vi "OLD_XLIN1.7-2048SQ TE0_Target.vi"() -> ()   [LabVIEW 2018]
uses:
  <vilib>/Platform/TimedLoop/XDataNode/timing_clust.ctl
  <vilib>/Platform/TimedLoop/XDataNode/nitl_modes.ctl
  <vilib>/Platform/TimedLoop/XDataNode/wakeup.ctl
  <vilib>/rvi/eio/common/nirviEmuTemplateMethod_errors.vi
  <vilib>/rvi/Emulation/niFpgaGetClockAttributes.vi
  <vilib>/rvi/Emulation/niFpgaSctlEmulationGetInTimedLoop.vi
  <vilib>/rvi/Emulation/niFpgaEmulationReportErrorSimple.vi
  <vilib>/rvi/Emulation/niFpgaProcessEmulError.vi
  <vilib>/rvi/Emulation/niFpgaCriticalErrorInLSC.vi
  <vilib>/rvi/interface/RandomDataEmulation/niFpgaRandomDataHandleErrors.vi
  <vilib>/eio/EIONode/EIONode.xnode
  <vilib>/Platform/TimedLoop/XDataNode/XDataNode.xnode
  <vilib>/rvi/DataTransferAndStorage/Container/XNode/niFpgaContainer.xnode
  <vilib>/rvi/interface/RandomDataEmulation/nirviRandomDataFpgaReadWriteTemplate.vi
  <vilib>/Platform/TimedLoop/XDataNode/XDNodeRunTimeDep.lvlib
panel:
  in  "Supply Select":u8(ring) items=["Local", "External"]
  in  "Falling CLK_3 = 1":u8=1
  in  "Rising CLK_4 = 2":u8=2
  in  "Counter R&F CLK_2 = 4":u8=4
  in  "F(F)/R(T)_FIFO":bool=TRUE
  in  "F(F)/R(T)_CmAD":bool
  in  "Falling CLK_7 = 1":u8=1
  in  "Rising CLK_7 = 1":u8=1
  in  "Falling CLK_6 = 2":u8=2
  in  "Rising CLK_6 = 2":u8=2
  in  "Counter R&F CLK_1 = 7":u8=7
  in  "Falling CLK_4 = 3":u8=3
  in  "Rising CLK_3 = 1":u8=1
  in  "Falling CLK_5 = 2":u8=2
  in  "Rising CLK_5 = 2":u8=2
  in  "Falling CLK_2 = 2":u8=2
  in  "Rising CLK_2 = 1":u8=1
  in  "Falling CLK_1 = 1":u8=1
  in  "Rising CLK_1 = 0":u8
  in  "Counter R CLK = 2":u8=2
  in  "ResetSetReg":bool
  in  "ResetSendData":bool
  out "SetRegIsDone":bool
  in  "Этап прошивки":T1(ring)
  in  "ResetFIFO":bool
  in  "Data Sample End":u8[](array[numeric])=[0, 5, 1, 0, 0]
  in  "Command End Readout":u8[](array[numeric])=[8, 4, 2, 0, 0]
  in  "Data Sample Start":u8[](array[numeric])=[0, 0, 1, 11, 1, 0, 0, 0, 0, 6, 0, 0, 15, 0, 1, 1, 5, 13, 13, 0]
  in  "Command Start Readout":u8[](array[numeric])=[8, 4, 2, 2, 2, 2, 9, 2, 2, 2, 2, 2, 2, 1, 1, 1, 1, 1, 1, 0]
  in  "Data Hold":u8[](array[numeric])=[0, 0, 0, 1, 1, 0, 0, 0, 5, 1, 0, 0, 0, 0, 0, 0, 0, 0, 0, 0, 3, 1, 0, 0, 1, 5, 1, 0, 0, 1, 3, 1, 0, 0, 1, 3, 1, 0, 0, 1, 11, 1, 11, 0, 1, 11, 1, 3, 0, 0, 0]
  in  "Command Start Integration":u8[](array[numeric])=[8, 4, 2, 2, 2, 2, 9, 2, 2, 2, 2, 2, 0, 0, 0, 0, 0, 8, 4, 2, 2, 2, 2, 9, 2, 2, 2, 2, 9, 2, 2, 2, 2, 9, 2, 2, 2, 2, 9, 2, 2, 2, 2, 9, 2, 2, 2, 2, 9, 0, 0]
  in  "SetReg":bool
  in  "Data Reset":u8[](array[numeric])=[0, 0, 0, 5, 0, 0, 0, 0, 0]
  in  "Command Reset":u8[](array[numeric])=[8, 4, 2, 2, 2, 2, 9, 0, 0]
  in  "IN1":bool
  in  "IN2":bool
  in  "RS":bool
  in  "1032 pixels":u16=1032
  out "FIFOIsDone":bool
  in  "R ADCCLK = 5":u16=5
  in  "R MCLK = 2":u16=2
  in  "FrameToFIFO":bool
  in  "Command array":bool[](array[boolean])=[FALSE, FALSE, FALSE, FALSE, FALSE, FALSE, FALSE, FALSE, FALSE, FALSE, FALSE, FALSE, FALSE, FALSE, FALSE, FALSE, FALSE]
  in  "Read(T)/Write(F)":bool
  in  "Enum":T2(ring)=enum."GREEN PGA"
  in  "Write Data":bool[](array[boolean])=[FALSE, FALSE, FALSE, FALSE, FALSE, FALSE, FALSE, FALSE, FALSE]
  out "READ":bool[](array[boolean])
  in  "Конфигурация":bool
  out "SendDataIsDone":bool
  in  "NumberOfAddFIFO":u16=2064
  in  "7..0(F)/0..7(T)":bool
  out "FIFOCounter":u16
  in  "CSTop":bool
  in  "ArraySize":u8=51
  in  "Command":u8[](array[numeric])=[8, 4, 2, 2, 2, 2, 2, 2, 2, 2, 2, 2, 2, 2, 2, 2, 2, 2, 2, 2, 2, 2, 2, 2, 2, 2, 2, 2, 2, 2, 2, 2, 2, 8, 4, 1, 1, 1, 1, 1, 1, 1, 1, 1, 0, 0, 0, 0, 0, 0, 0]
  in  "Data":u8[](array[numeric])=[0, 9, 12, 11, 0, 6, 0, 2, 11, 0, 8, 0, 0, 0, 0, 9, 1, 3, 3, 7, 15, 15, 5, 15, 0, 1, 15, 15, 5, 8, 5, 2, 3, 0, 8, 2, 3, 3, 3, 3, 3, 3, 3, 2, 0, 0, 0, 0, 0, 0, 0]
  in  "Data CSBot":u8[](array[numeric])=[0, 9, 8, 11, 0, 6, 0, 2, 11, 0, 8, 0, 0, 0, 0, 9, 1, 3, 11, 7, 15, 15, 5, 15, 0, 1, 15, 15, 5, 8, 5, 2, 3, 0, 8, 2, 3, 3, 3, 3, 3, 3, 3, 2, 0]
  in  "CSBot":bool
  in  "Автомат":bool
  in  "Data CSTop":u8[](array[numeric])=[0, 9, 12, 11, 0, 6, 0, 2, 11, 0, 8, 0, 0, 0, 0, 9, 1, 3, 3, 7, 15, 15, 5, 15, 0, 1, 15, 15, 5, 8, 5, 2, 3, 0, 8, 2, 3, 3, 3, 3, 3, 3, 3, 2, 0]
  in  "Command CS":u8[](array[numeric])=[8, 4, 2, 2, 2, 2, 2, 2, 2, 2, 2, 2, 2, 2, 2, 2, 2, 2, 2, 2, 2, 2, 2, 2, 2, 2, 2, 2, 2, 2, 2, 2, 2, 8, 4, 1, 1, 1, 1, 1, 1, 1, 1, 1, 0]
  in  "Stop_FPGA":bool
  in  "SendData":bool
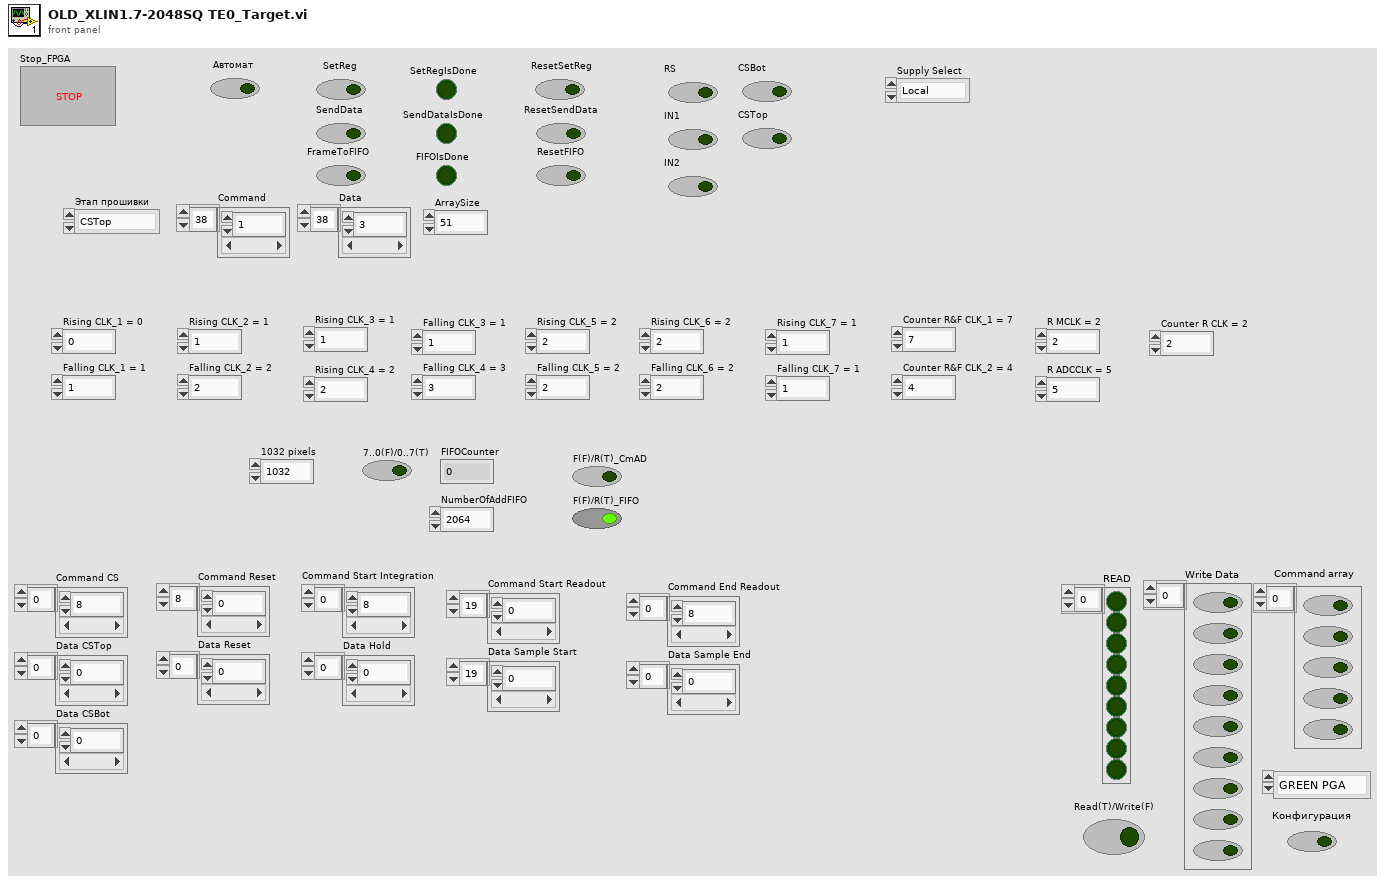
[diagram p1: front panel]
types:
  T1 = enum16{"CSTop", "CSBot", "Reset", "Hold", "Sample Start", "Sample End"}
  T2 = enum16{"Configuration", "MUX", "RED PGA", "GREEN PGA", "BLUE PGA", "RED OFF", "GREEN OFF", "BLUE OFF"}
  T3 = typedef "XDNodeRunTimeDep.lvlib/timing_clust.ctl" = cluster{"Expected End [f-1]":u64, "Actual End [f-1]":u64, "Finished Late? [f-1]":bool, "Expected End [i-1]":u64, "Actual End [i-1]":u64, "Finished Late? [i-1]":bool, "Expected Start [i]":u64, "Actual Start [i]":u64, "Expected Start [f]":u64, "Actual Start [f]":u64, "Source Name":string, "Structure Name":string, "Period":i64, "Deadline":i64, "Offset":i64, "Start":i64, "Priority":i32, "Timeout":i32, "Mode":T4, "Wakeup Reason":T5, "Error":errorcluster, "Source Type":string, "Secondary Source Type":string, "Global End Time":u64, "Global Start Time":u64, "Frame Duration":u64, "Iteration Duration":u64, "Assigned CPU":i32, "I/O Scan Engine Mode":u32}
  T4 = typedef "XDNodeRunTimeDep.lvlib/nitl_modes.ctl" = enum32{"No Change", "Process missed periods, maintain original phase", "Discard missed periods, maintain original phase", "Process missed periods, ignore original phase", "Discard missed periods, ignore original phase"}
  T5 = typedef "XDNodeRunTimeDep.lvlib/wakeup.ctl" = enum32{"Normal", "Aborted", "Asynchronous wakeup", "Timing source error", "Timed loop error", "Timeout"}
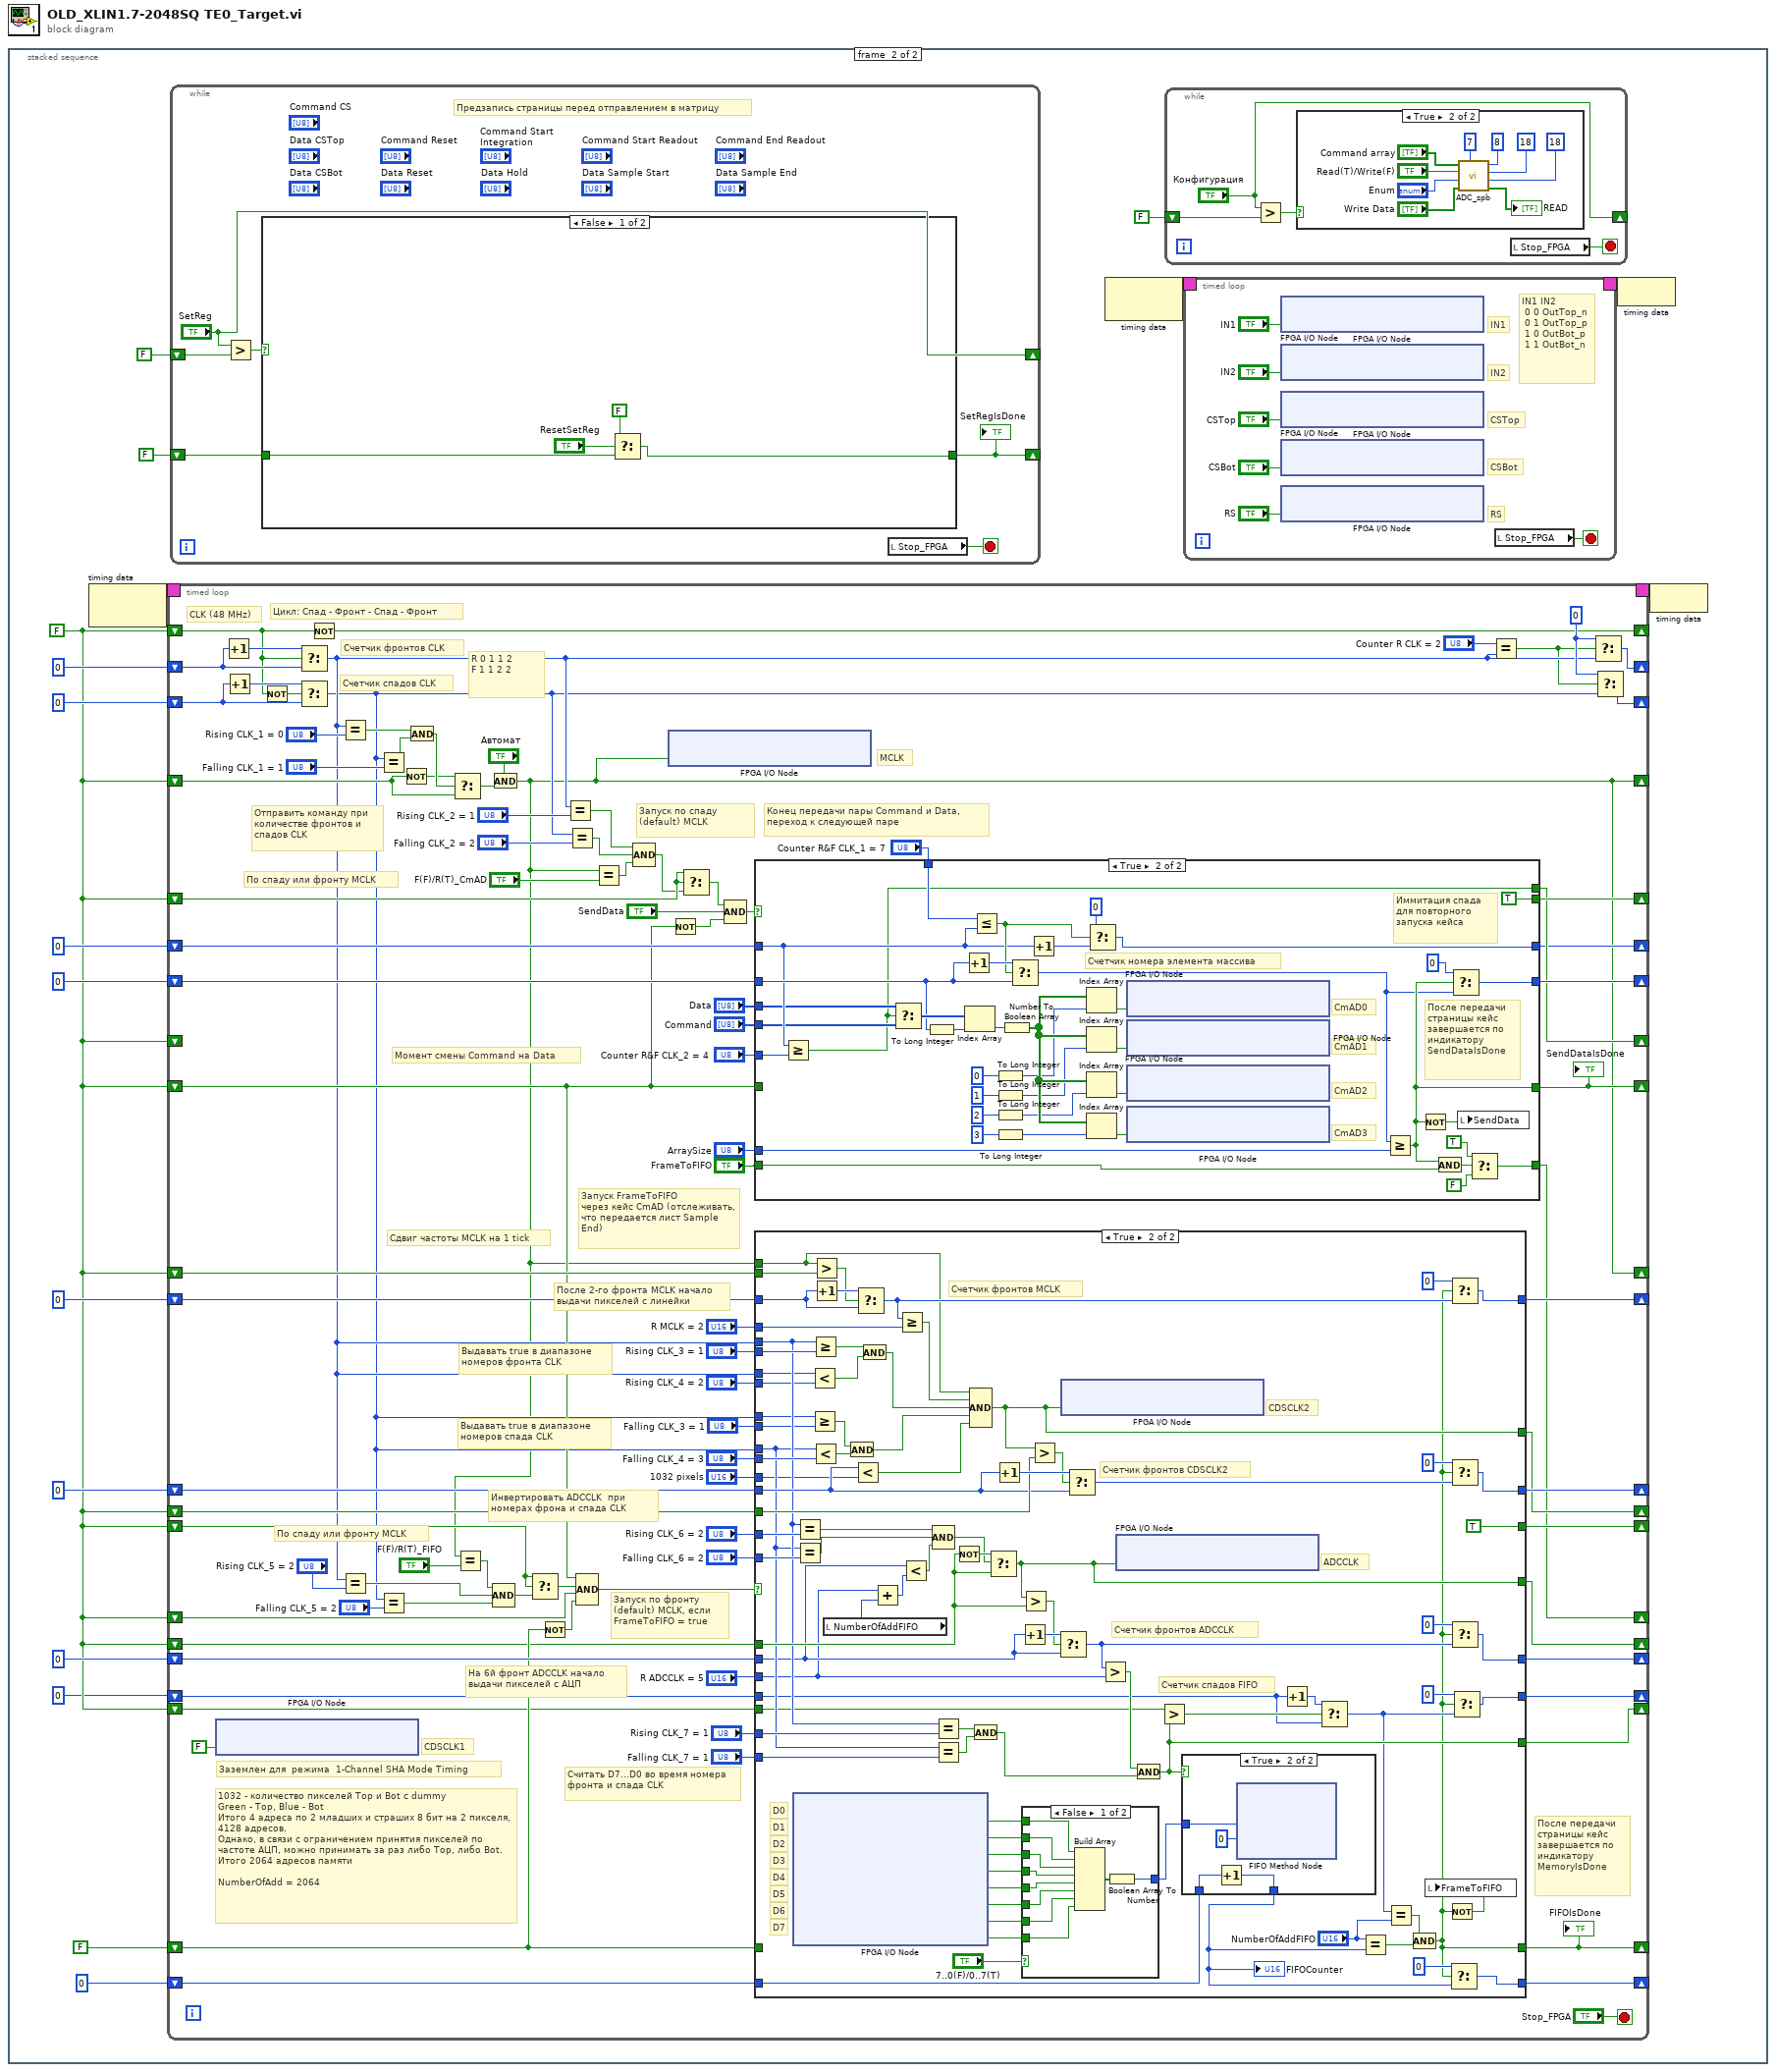
[diagram p0: block diagram]
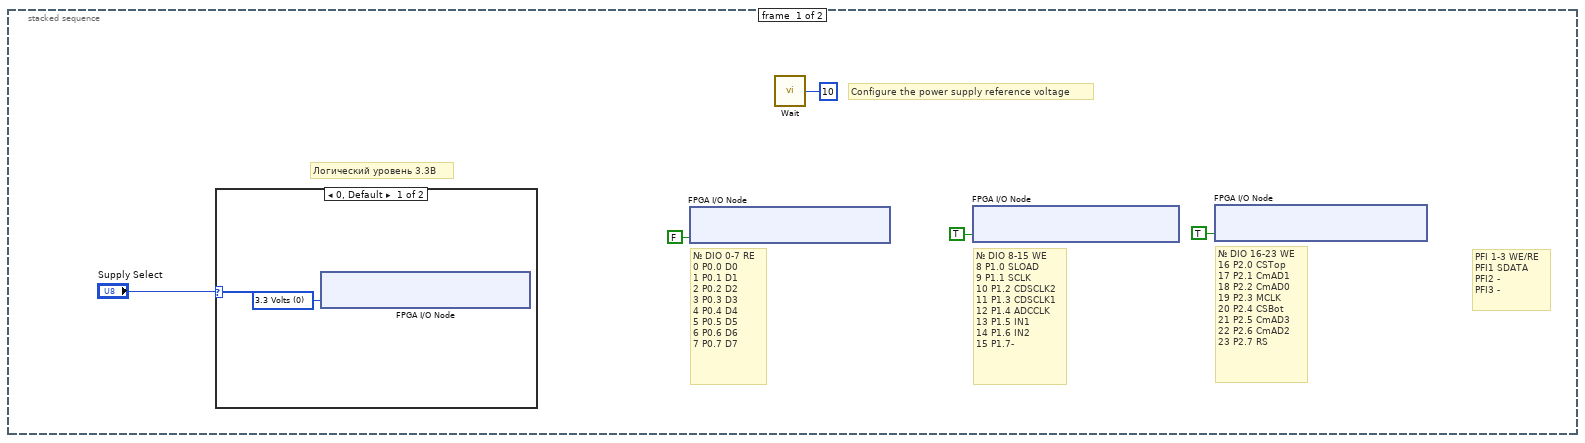
[diagram p2: hidden frame]
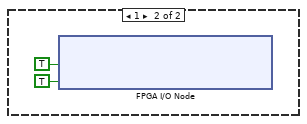
[diagram p3: hidden frame]
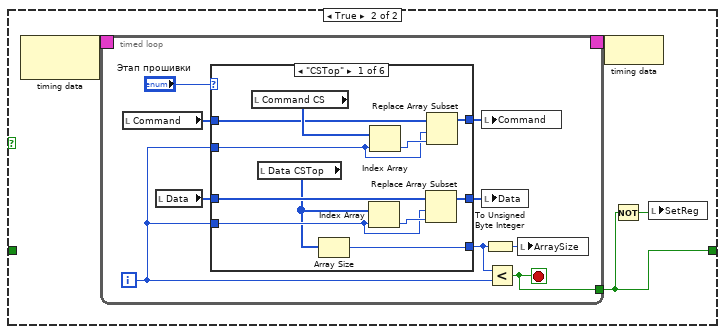
[diagram p4: hidden frame]
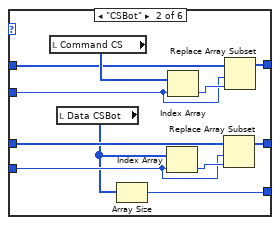
[diagram p5: hidden frame]
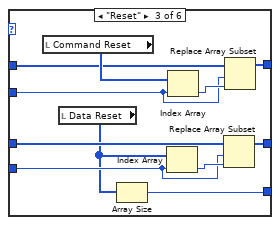
[diagram p6: hidden frame]
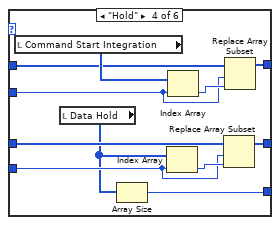
[diagram p7: hidden frame]
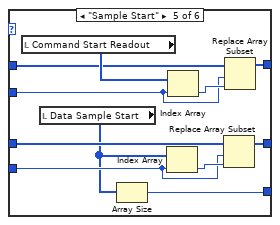
[diagram p8: hidden frame]
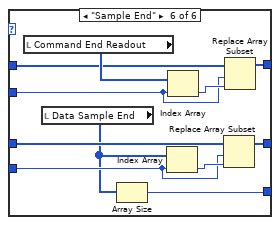
[diagram p9: hidden frame]
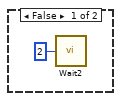
[diagram p10: hidden frame]
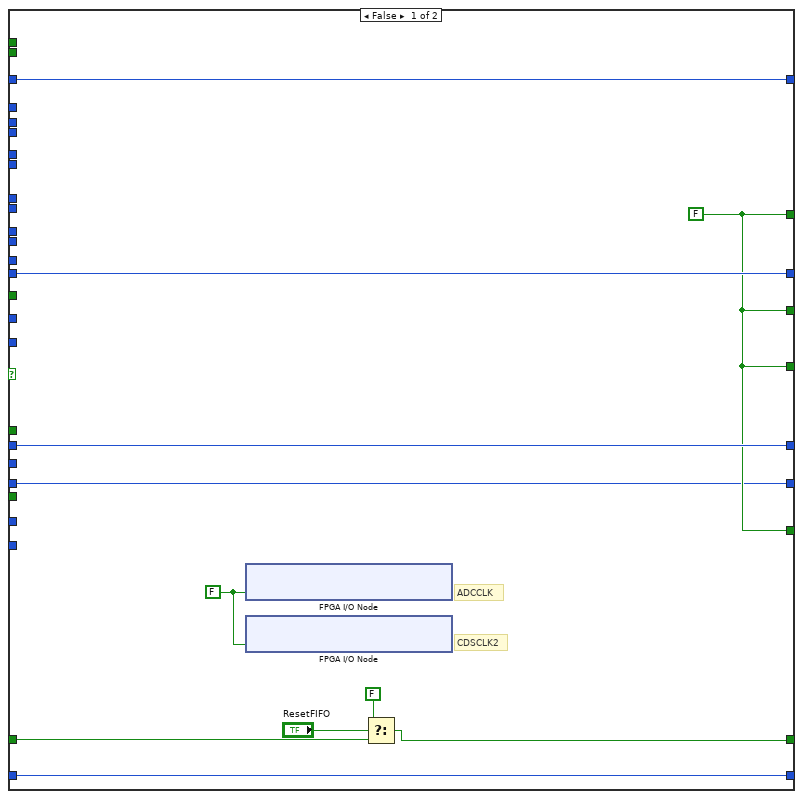
[diagram p11: hidden frame]
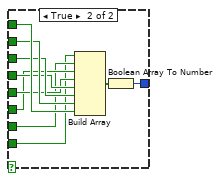
[diagram p12: hidden frame]
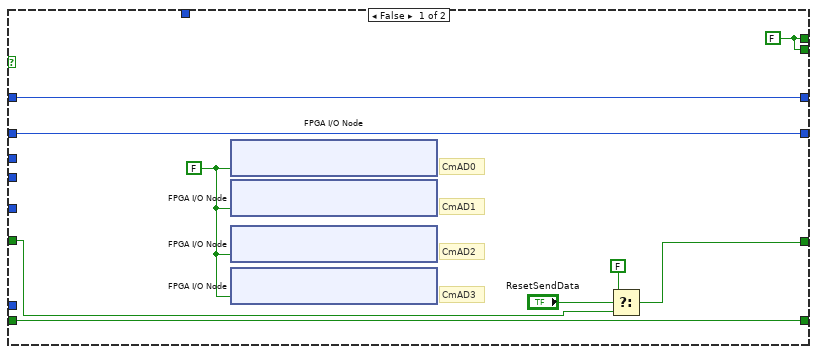
[diagram p14: hidden frame]
diagram:
  n1 = stacked-sequence {
    frame #0 {
      # "Логический уровень 3.3В"
      # "№\tDIO 16-23\tWE\n16\tP2.0\tCSTop\n17\tP2.1\tCmAD1\n18\tP2.2\tCmAD0\n19\tP2.3\tMCLK\n20\tP2.4\tCSBot\n21\tP2.5\tCmAD3\n22\tP2.6\tCmAD2\n23\tP2.7\tRS"
      # "№\tDIO 8-15\tWE\n8\tP1.0\tSLOAD\n9\tP1.1\tSCLK\n10\tP1.2\tCDSCLK2\n11\tP1.3\tCDSCLK1\n12\tP1.4\tADCCLK\n13\tP1.5\tIN1\n14\tP1.6\tIN2\n15\tP1.7-"
      # "PFI 1-3\tWE/RE\nPFI1\tSDATA\nPFI2\t-\nPFI3\t-"
      # "№\tDIO 0-7\tRE\n0\tP0.0\tD0\n1\tP0.1\tD1\n2\tP0.2\tD2\n3\tP0.3\tD3\n4\tP0.4\tD4\n5\tP0.5\tD5\n6\tP0.6\tD6\n7\tP0.7\tD7"
      # "Configure the power supply reference voltage"
      n2 = case shown="0, Default" "Supply Select" {
        frame 0, Default {
          w6 = u8 0 items=["3.3 Volts", "2.5 Volts", "1.8 Volts"] ("Internal Power Supply Voltage")
          n3 = xnode "FPGA I/O Node"("IO Module\\Local_Supply_Select"=w6) -> ()  [unwired: 1 in, 1 out]
        }
        frame 1 {
          n4 = xnode "FPGA I/O Node"("IO Module\\DDCA_Supply_Select"=TRUE ("IO Module\\DDCA_Supply_Select"), "IO Module\\DDCB_Supply_Select"=TRUE ("IO Module\\DDCB_Supply_Select")) -> ()  [unwired: 2 in, 2 out]
        }
      }
      n5 = xnode "FPGA I/O Node"("IO Module\\DDCA_DIO0-7_WE"=FALSE ("IO Module\\DDCA_DIO0-7_WE")) -> ()  [unwired: 1 in, 1 out]
      n6 = call "Wait"("Count(mSec)"=u8 10) -> ()  [unwired: 1 out]
      n7 = xnode "FPGA I/O Node"("IO Module\\DDCA_DIO8-15_WE"=TRUE ("IO Module\\DDCA_DIO8-15_WE")) -> ()  [unwired: 1 in, 1 out]
      n8 = xnode "FPGA I/O Node"("IO Module\\DDCA_DIO16-23_WE"=TRUE ("IO Module\\DDCA_DIO16-23_WE")) -> ()  [unwired: 1 in, 1 out]
    }
    frame #1 {
      w10 = FALSE
      n9 = node-c288() -> (w26:T3)  [unwired: 1 in]
      n10 = timed-loop {
        timing: w26 -> [_]
        timing-out: [_] -> w25
        shift-right: [w146] -> _
        shift-left: w10 -> [w209]
        shift-right: [w235] -> _
        shift-left: u8 0 -> [w239]
        shift-right: [w234] -> _
        shift-left: w10 -> [w220]
        shift-right: [w233] -> _
        shift-left: u16 0 -> [w232]
        shift-right: [w230] -> _
        shift-left: u16 0 -> [w231]
        shift-right: [w228] -> _
        shift-left: u16 0 -> [w229]
        shift-right: [w226] -> _
        shift-left: u16 0 -> [w227]
        shift-right: [w225] -> _
        shift-left: w10 -> [w176]
        shift-right: [w224] -> _
        shift-left: FALSE ("IO Module\\DDCA_DIO11_Write") -> [w212]
        shift-right: [w153] -> _
        shift-left: w10 -> [w152]
        shift-right: [w223] -> _
        shift-left: w10 -> [w163]
        shift-right: [w217] -> _
        shift-left: w10 -> [w218]
        shift-right: [w213] -> _
        shift-left: w10 -> [w172]
        shift-right: [w205] -> _
        shift-left: u8 0 -> [w198]
        shift-right: [w206] -> _
        shift-left: u8 0 -> [w199]
        shift-right: [w184] -> _
        shift-left: w10 -> [_]
        shift-right: [w182] -> _
        shift-left: u8 0 -> [w183]
        shift-right: [w146] -> _
        shift-left: w10 -> [w180]
        shift-right: [w171] -> _
        shift-left: w10 -> [w173]
        shift-right: [w159] -> _
        shift-left: w10 -> [w160]
        shift-right: [w157] -> _
        shift-left: u16 0 -> [w158]
        stop <- "Stop_FPGA" stop-if-true
        w204 = u8 0 ("f")
        # "Цикл: Спад - Фронт - Спад - Фронт"
        # "Конец передачи пары Command и Data, переход к следующей паре"
        # "Запуск по спаду (default) MCLK"
        # "Момент смены Command на Data"
        # "По спаду или фронту MCLK"
        # "Считать D7...D0 во время номера фронта и спада CLK"
        # "Инвертировать ADCCLK  при номерах фрона и спада CLK"
        # "Выдавать true в диапазоне номеров спада CLK"
        # "Выдавать true в диапазоне номеров фронта CLK"
        # "По спаду или фронту MCLK"
        # "Заземлен для  режима  1-Channel SHA Mode Timing"
        # "CDSCLK1"
        # "R 0 1 1 2\nF 1 1 2 2"
        # "Счетчик спадов CLK"
        # "Счетчик фронтов CLK"
        # "После 2-го фронта MCLK начало выдачи пикселей с линейки"
        # "На 6й фронт ADCCLK начало выдачи пикселей с АЦП"
        # "Отправить команду при количестве фронтов и спадов CLK"
        # "После передачи страницы кейс завершается по индикатору MemoryIsDone"
        # "Запуск FrameToFIFO\nчерез кейс CmAD (отслеживать, что передается лист Sample End)"
        # "CLK (48 MHz)"
        # "1032 - количество пикселей Top и Bot с dummy\nGreen - Top, Blue - Bot\nИтого 4 адреса по 2 младших и страших 8 бит на 2 пикселя, 4128 адресов.\nОднако, в связи с ограничением принятия пикселей по частоте АЦП, можно принимать за раз либо Top, либо Bot. Итого 2064 адресов памяти\n\nNumberOfAdd = 2064"
        # "Сдвиг частоты MCLK на 1 tick"
        # "Запуск по фронту (default) MCLK, если FrameToFIFO = true"
        # "MCLK"
        n11 = xnode "FPGA I/O Node"("IO Module\\DDCA_DIO11_Write"=FALSE ("IO Module\\DDCA_DIO11_Write")) -> ()  [unwired: 1 in, 1 out]
        n12 = Increment(x=w199) -> (x+1=w208:u8)
        n13 = Increment(x=w198) -> (x+1=w207:u8)
        n14 = Not(x=w152) -> (.not. x?=w210:bool)
        n15 = Select(t=w208, s=w152, f=w199) -> (s? t:f=w150:u8)
        n16 = Select(t=w207, s=w210, f=w198) -> (s? t:f=w149:u8)
        n17 = Not(x=w152) -> (.not. x?=w153:bool)
        n18 = Equal?(x=w150, y="Rising CLK_1 = 0") -> (x = y?=w203:bool)
        n19 = Equal?(x=w150, y="Rising CLK_5 = 2") -> (x = y?=w179:bool)
        n20 = Equal?(x=w149, y="Falling CLK_1 = 1") -> (x = y?=w200:bool)
        n21 = Equal?(x=w149, y="Falling CLK_5 = 2") -> (x = y?=w178:bool)
        n22 = Not(x=w209) -> (.not. x?=w147:bool)
        n23 = And(x=w203, y=w200) -> (x .and. y?=w197:bool)
        n24 = Select(t=w147, s=w197, f=w209) -> (s? t:f=w222:bool)
        n25 = And(x="Автомат", y=w222) -> (x .and. y?=w146:bool)
        n26 = Equal?(x=w146, y="F(F)/R(T)_FIFO") -> (x = y?=w165:bool)
        n27 = Compound Arithmetic op=AND(w165, w179, w178) -> (w177:bool)
        n28 = Select(t=w218, s=w218, f=w177) -> (s? t:f=w162:bool)
        n29 = Not(x=w212) -> (.not. x?=w170:bool)
        n30 = Equal?(x=w150, y="Rising CLK_2 = 1") -> (x = y?=w189:bool)
        n31 = Equal?(x=w149, y="Falling CLK_2 = 2") -> (x = y?=w188:bool)
        n32 = Compound Arithmetic op=AND(w163, w162, w172, w170) -> (w219:bool)
        n33 = Equal?(x=w146, y="F(F)/R(T)_CmAD") -> (x = y?=w187:bool)
        n34 = Compound Arithmetic op=AND(w189, w188, w187) -> (w144:bool)
        n35 = xnode "FPGA I/O Node"("IO Module\\DDCA_DIO19_Write"=w146) -> ()  [unwired: 1 in, 1 out]
        n36 = Not(x=w163) -> (.not. x?=w216:bool)
        n37 = Select(t=w220, s=w220, f=w144) -> (s? t:f=w221:bool)
        n38 = Compound Arithmetic op=AND(w221, "SendData", w216) -> (w145:bool)
        n39 = case shown="True" w145 {
          tunnel: w239 -> [w365 w388]
          tunnel: "ArraySize" -> [_ w387]
          tunnel: [w365 w384] -> w235
          tunnel: "FrameToFIFO" -> [w366 w400]
          tunnel: [w363 TRUE] -> w234
          tunnel: [w367 w383] -> w223
          tunnel: w163 -> [w368 _]
          tunnel: [w366 w385] -> w213
          tunnel: "Command" -> [_ w373]
          tunnel: "Data" -> [_ w372]
          tunnel: [w363 w371] -> w184
          tunnel: w183 -> [w364 w374]
          tunnel: [w364 w377] -> w182
          tunnel: "Counter R&F CLK_1 = 7" -> [_ w378]
          tunnel: "Counter R&F CLK_2 = 4" -> [_ w375]
          frame False {
            w362 = FALSE ("t")
            w363 = FALSE
            # "CmAD3"
            # "CmAD2"
            # "CmAD1"
            # "CmAD0"
            n40 = xnode "FPGA I/O Node"("IO Module\\DDCA_DIO18_Write"=w362) -> ()  [unwired: 1 in, 1 out]
            n41 = xnode "FPGA I/O Node"("IO Module\\DDCA_DIO17_Write"=w362) -> ()  [unwired: 1 in, 1 out]
            n42 = xnode "FPGA I/O Node"("IO Module\\DDCA_DIO22_Write"=w362) -> ()  [unwired: 1 in, 1 out]
            n43 = xnode "FPGA I/O Node"("IO Module\\DDCA_DIO21_Write"=w362) -> ()  [unwired: 1 in, 1 out]
            n44 = Select(t=FALSE, s="ResetSendData", f=w368) -> (s? t:f=w367:bool)
          }
          frame True {
            # "Иммитация спада для повторного запуска кейса"
            # "После передачи страницы кейс завершается по индикатору SendDataIsDone"
            # "Счетчик номера элемента массива"
            # "CmAD3"
            # "CmAD2"
            # "CmAD1"
            # "CmAD0"
            n45 = Greater Or Equal?(x=w374, y=w375) -> (x >= y?=w371:bool)
            n46 = Select(t=w372, s=w371, f=w373) -> (s? t:f=w408:u8[])
            n47 = To Long Integer(number=w388) -> (32bit integer=w407:i32)
            n48 = Increment(x=w388) -> (x+1=w410:u8)
            n49 = Index Array(array=w408, index=w407) -> (element=w409:u8)
            n50 = Less Or Equal?(x=w378, y=w374) -> (x <= y?=w380:bool)
            n51 = To Long Integer(number=u8 0 ("CmAD0_bit_0")) -> (32bit integer=w393:i32)
            n52 = To Long Integer(number=u8 1 ("CmAD1_bit_1")) -> (32bit integer=w392:i32)
            n53 = To Long Integer(number=u8 2 ("CmAD2_bit_2")) -> (32bit integer=w391:i32)
            n54 = To Long Integer(number=u8 3 ("CmAD3_bit_3")) -> (32bit integer=w389:i32)
            n55 = Number To Boolean Array(number=w409) -> (Boolean array=w405:bool[])
            n56 = Select(t=w410, s=w380, f=w388) -> (s? t:f=w382:u8)
            n57 = Increment(x=w374) -> (x+1=w376:u8)
            n58 = Index Array(array=w405, index=w393) -> (element=w406:bool)
            n59 = Index Array(array=w405, index=w392) -> (element=w402:bool)
            n60 = Index Array(array=w405, index=w391) -> (element=w404:bool)
            n61 = Index Array(array=w405, index=w389) -> (element=w403:bool)
            n62 = Select(t=u8 0, s=w380, f=w376) -> (s? t:f=w377:u8)
            n63 = xnode "FPGA I/O Node"("IO Module\\DDCA_DIO18_Write"=w406) -> ()  [unwired: 1 in, 1 out]
            n64 = xnode "FPGA I/O Node"("IO Module\\DDCA_DIO17_Write"=w402) -> ()  [unwired: 1 in, 1 out]
            n65 = xnode "FPGA I/O Node"("IO Module\\DDCA_DIO22_Write"=w404) -> ()  [unwired: 1 in, 1 out]
            n66 = xnode "FPGA I/O Node"("IO Module\\DDCA_DIO21_Write"=w403) -> ()  [unwired: 1 in, 1 out]
            n67 = Greater Or Equal?(x=w382, y=w387) -> (x >= y?=w383:bool)
            n68 = Not(x=w383) -> (.not. x?=w386:bool)
            n69 = And(x=w383, y=w400) -> (x .and. y?=w401:bool)
            n70 = Select(t=u8 0, s=w383, f=w382) -> (s? t:f=w384:u8)
            n71 = local write "SendData"(w386) -> ()
            n72 = Select(t=TRUE ("f"), s=w401, f=FALSE) -> (s? t:f=w385:bool)
          }
        }
        "SendDataIsDone" <- w223
        n73 = case shown="True" w219 {
          tunnel: [w246 w254] -> w233
          tunnel: w232 -> [w246 w326]
          tunnel: w231 -> [w244 w336]
          tunnel: [w244 w315] -> w230
          tunnel: w229 -> [w243 w281]
          tunnel: [w243 w308] -> w228
          tunnel: w227 -> [w245 w317]
          tunnel: [w245 w313] -> w226
          tunnel: w180 -> [_ w303]
          tunnel: w176 -> [_ w318]
          tunnel: [w241 w285] -> w225
          tunnel: [w248 w251] -> w224
          tunnel: w212 -> [w247 _]
          tunnel: [w241 TRUE ("f")] -> w217
          tunnel: "R MCLK = 2" -> [_ w283]
          tunnel: "1032 pixels" -> [_ w282]
          tunnel: "R ADCCLK = 5" -> [_ w278]
          tunnel: w150 -> [_ w292]
          tunnel: "Rising CLK_3 = 1" -> [_ w306]
          tunnel: w149 -> [_ w291]
          tunnel: "Falling CLK_4 = 3" -> [_ w305]
          tunnel: w146 -> [_ w261]
          tunnel: "Rising CLK_6 = 2" -> [_ w302]
          tunnel: "Falling CLK_6 = 2" -> [_ w301]
          tunnel: w173 -> [_ w298]
          tunnel: [w241 w284] -> w171
          tunnel: "Rising CLK_7 = 1" -> [_ w293]
          tunnel: "Falling CLK_7 = 1" -> [_ w294]
          tunnel: w160 -> [_ w276]
          tunnel: [w241 w275] -> w159
          tunnel: w158 -> [w240 w272]
          tunnel: [w240 w270] -> w157
          tunnel: "Rising CLK_4 = 2" -> [_ w264]
          tunnel: w150 -> [_ w263]
          tunnel: w149 -> [_ w256]
          tunnel: "Falling CLK_3 = 1" -> [_ w255]
          frame False {
            w242 = FALSE ("IO Module\\DDCA_DIO12_Write")
            w241 = FALSE
            # "CDSCLK2"
            # "ADCCLK"
            n74 = xnode "FPGA I/O Node"("IO Module\\DDCA_DIO12_Write"=w242) -> ()  [unwired: 1 in, 1 out]
            n75 = xnode "FPGA I/O Node"("IO Module\\DDCA_DIO10_Write"=w242) -> ()  [unwired: 1 in, 1 out]
            n76 = Select(t=FALSE, s="ResetFIFO", f=w247) -> (s? t:f=w248:bool)
          }
          frame True {
            # "Счетчик спадов FIFO"
            # "ADCCLK"
            # "Счетчик фронтов CDSCLK2"
            # "Счетчик фронтов ADCCLK"
            # "Счетчик фронтов MCLK"
            # "D7"
            # "D6"
            # "D5"
            # "D4"
            # "D3"
            # "D2"
            # "D1"
            # "D0"
            # "CDSCLK2"
            n77 = xnode "FPGA I/O Node"() -> ("IO Module\\DDCA_DIO0_Read"=w327:bool, "IO Module\\DDCA_DIO1_Read"=w328:bool, "IO Module\\DDCA_DIO2_Read"=w329:bool, "IO Module\\DDCA_DIO3_Read"=w330:bool, "IO Module\\DDCA_DIO4_Read"=w331:bool, "IO Module\\DDCA_DIO5_Read"=w332:bool, "IO Module\\DDCA_DIO6_Read"=w333:bool, "IO Module\\DDCA_DIO7_Read"=w334:bool)  [unwired: 8 in, 8 out]
            n78 = Equal?(x=w292, y=w302) -> (x = y?=w287:bool)
            n79 = Equal?(x=w291, y=w301) -> (x = y?=w289:bool)
            n80 = Less?(x=w263, y=w264) -> (x < y?=w262:bool)
            n81 = Greater Or Equal?(x=w256, y=w255) -> (x >= y?=w258:bool)
            n82 = Greater Or Equal?(x=w292, y=w306) -> (x >= y?=w265:bool)
            n83 = Less?(x=w291, y=w305) -> (x < y?=w304:bool)
            n84 = Greater?(x=w261, y=w303) -> (0:w321:bool)
            n85 = Increment(x=w336) -> (x+1=w324:u16)
            n86 = local read "NumberOfAddFIFO"() -> (w279:u16)
            n87 = And(x=w258, y=w304) -> (x .and. y?=w257:bool)
            n88 = Less?(x=w317, y=w282) -> (x < y?=w290:bool)
            n89 = Select(t=w324, s=w321, f=w336) -> (s? t:f=w286:u16)
            n90 = And(x=w265, y=w262) -> (x .and. y?=w259:bool)
            n91 = Add(x=w278, y=w279) -> (x+y=w277:u16)
            n92 = Greater Or Equal?(x=w286, y=w283) -> (x >= y?=w260:bool)
            n93 = Less?(x=w281, y=w277) -> (x < y?=w280:bool)
            n94 = Compound Arithmetic op=AND(w287, w289, w280) -> (w288:bool)
            n95 = Equal?(x=w292, y=w293) -> (x = y?=w297:bool)
            n96 = Equal?(x=w291, y=w294) -> (x = y?=w296:bool)
            n97 = Not(x=w298) -> (.not. x?=w300:bool)
            n98 = Compound Arithmetic op=AND(w261, w260, w259, w257, w290) -> (w285:bool)
            n99 = And(x=w297, y=w296) -> (x .and. y?=w295:bool)
            n100 = Select(t=w300, s=w288, f=w298) -> (s? t:f=w284:bool)
            n101 = Increment(x=w317) -> (x+1=w322:u16)
            n102 = Increment(x=w281) -> (x+1=w323:u16)
            n103 = Greater?(x=w284, y=w298) -> (0:w299:bool)
            n104 = case shown="False" "7..0(F)/0..7(T)" {
              tunnel: w327 -> [w346 w354]
              tunnel: w328 -> [w345 w353]
              tunnel: w329 -> [w344 w352]
              tunnel: w330 -> [w343 w351]
              tunnel: w331 -> [w342 w350]
              tunnel: w332 -> [w341 w349]
              tunnel: w333 -> [w340 w348]
              tunnel: w334 -> [w339 w347]
              tunnel: [w337 w355] -> w325
              frame False {
                n105 = Build Array(w346, w345, w344, w343, w342, w341, w340, w339) -> (w338:bool[])
                n106 = Boolean Array To Number(Boolean array=w338) -> (number=w337:u8)
              }
              frame True {
                n107 = Build Array(w347, w348, w349, w350, w351, w352, w353, w354) -> (w356:bool[])
                n108 = Boolean Array To Number(Boolean array=w356) -> (number=w355:u8)
              }
            }
            n109 = Greater?(x=w285, y=w318) -> (0:w319:bool)
            n110 = Select(t=w323, s=w299, f=w281) -> (s? t:f=w307:u16)
            n111 = xnode "FPGA I/O Node"("IO Module\\DDCA_DIO10_Write"=w285) -> ()  [unwired: 1 in, 1 out]
            n112 = Select(t=w322, s=w319, f=w317) -> (s? t:f=w312:u16)
            n113 = Greater?(x=w307, y=w278) -> (0:w320:bool)
            n114 = xnode "FPGA I/O Node"("IO Module\\DDCA_DIO12_Write"=w284) -> ()  [unwired: 1 in, 1 out]
            n115 = And(x=w320, y=w295) -> (x .and. y?=w275:bool)
            n116 = Greater?(x=w276, y=w275) -> (0:w274:bool)
            n117 = case shown="True" w275 {
              tunnel: [w357 w361] -> w253
              tunnel: w326 -> [w357 w360]
              tunnel: w325 -> [_ w358]
              frame False {
              }
              frame True {
                n118 = Increment(x=w360) -> (x+1=w361:u16)
                n119 = xnode ("FIFO Method Node")("Element"=w358, "Timeout"=0) -> ()  [unwired: 1 in, 2 out]
              }
            }
            "FIFOCounter" <- w253
            n120 = Increment(x=w272) -> (x+1=w273:u16)
            n121 = Select(t=w273, s=w274, f=w272) -> (s? t:f=w268:u16)
            n122 = Equal?(x="NumberOfAddFIFO", y=w253) -> (x = y?=w266:bool)
            n123 = Equal?(x=w268, y="NumberOfAddFIFO") -> (x = y?=w269:bool)
            n124 = Compound Arithmetic op=AND(w269, w266) -> (w251:bool)
            n125 = Not(x=w251) -> (.not. x?=w252:bool)
            n126 = local write "FrameToFIFO"(w252) -> ()
            n127 = Select(t=u16 0, s=w251, f=w253) -> (s? t:f=w254:u16)
            n128 = Select(t=u16 0, s=w251, f=w286) -> (s? t:f=w315:u16)
            n129 = Select(t=u16 0, s=w251, f=w312) -> (s? t:f=w313:u16)
            n130 = Select(t=u16 0, s=w251, f=w307) -> (s? t:f=w308:u16)
            n131 = Select(t=u16 0, s=w251, f=w268) -> (s? t:f=w270:u16)
          }
        }
        "FIFOIsDone" <- w224
        n132 = Equal?(x="Counter R CLK = 2", y=w150) -> (x = y?=w148:bool)
        n133 = Select(t=w204, s=w148, f=w150) -> (s? t:f=w206:u8)
        n134 = Select(t=w204, s=w148, f=w149) -> (s? t:f=w205:u8)
      }
      n135 = while {
        shift-right: ["SetReg"] -> _
        shift-left: FALSE -> [w41]
        shift-right: [w37] -> _
        shift-left: FALSE -> [w38]
        stop <- w42 stop-if-true
        # "Предзапись страницы перед отправлением в матрицу"
        n136 = Greater?(x="SetReg", y=w41) -> (0:w40:bool)
        n137 = case shown="False" w40 {
          tunnel: [w43 w47] -> w37
          tunnel: w38 -> [w45 _]
          frame False {
            n138 = Select(t=FALSE, s="ResetSetReg", f=w45) -> (s? t:f=w43:bool)
          }
          frame True {
            n139 = node-c288() -> (w50:T3)  [unwired: 1 in]
            n140 = timed-loop {
              timing: w50 -> [_]
              timing-out: [_] -> w49
              tunnel: [w53] -> w47
              i -> [w54]
              stop <- w53 stop-if-true
              n141 = local read "Command"() -> (w58:u8[])
              n142 = local read "Data"() -> (w57:u8[])
              n143 = case shown="\"CSTop\"" "Этап прошивки" {
                tunnel: w54 -> [w67 w78 w89 w100 w111 w122]
                tunnel: w58 -> [w66 w77 w88 w99 w110 w121]
                tunnel: w57 -> [w65 w76 w87 w98 w109 w120]
                tunnel: [w64 w75 w86 w97 w108 w119] -> w56
                tunnel: [w63 w74 w85 w96 w107 w118] -> w55
                tunnel: w54 -> [w62 w73 w84 w95 w106 w117]
                tunnel: [w60 w71 w82 w93 w104 w115] -> w51
                frame "CSTop" {
                  n144 = local read "Command CS"() -> (w69:u8[])
                  n145 = local read "Data CSTop"() -> (w61:u8[])
                  n146 = Array Size(array=w61) -> (size(s)=w60:i32)
                  n147 = Index Array(array=w61, index=w62) -> (element=w68:u8)
                  n148 = Index Array(array=w69, index=w67) -> (element=w70:u8)
                  n149 = Replace Array Subset(array=w65, new element=w68, index=w62) -> (w63:u8[])
                  n150 = Replace Array Subset(array=w66, new element=w70, index=w67) -> (w64:u8[])
                }
                frame "CSBot" {
                  n151 = local read "Command CS"() -> (w80:u8[])
                  n152 = local read "Data CSBot"() -> (w72:u8[])
                  n153 = Array Size(array=w72) -> (size(s)=w71:i32)
                  n154 = Index Array(array=w72, index=w73) -> (element=w79:u8)
                  n155 = Index Array(array=w80, index=w78) -> (element=w81:u8)
                  n156 = Replace Array Subset(array=w76, new element=w79, index=w73) -> (w74:u8[])
                  n157 = Replace Array Subset(array=w77, new element=w81, index=w78) -> (w75:u8[])
                }
                frame "Reset" {
                  n158 = local read "Command Reset"() -> (w91:u8[])
                  n159 = local read "Data Reset"() -> (w83:u8[])
                  n160 = Array Size(array=w83) -> (size(s)=w82:i32)
                  n161 = Index Array(array=w83, index=w84) -> (element=w90:u8)
                  n162 = Index Array(array=w91, index=w89) -> (element=w92:u8)
                  n163 = Replace Array Subset(array=w87, new element=w90, index=w84) -> (w85:u8[])
                  n164 = Replace Array Subset(array=w88, new element=w92, index=w89) -> (w86:u8[])
                }
                frame "Hold" {
                  n165 = local read "Command Start Integration"() -> (w102:u8[])
                  n166 = local read "Data Hold"() -> (w94:u8[])
                  n167 = Array Size(array=w94) -> (size(s)=w93:i32)
                  n168 = Index Array(array=w94, index=w95) -> (element=w101:u8)
                  n169 = Index Array(array=w102, index=w100) -> (element=w103:u8)
                  n170 = Replace Array Subset(array=w98, new element=w101, index=w95) -> (w96:u8[])
                  n171 = Replace Array Subset(array=w99, new element=w103, index=w100) -> (w97:u8[])
                }
                frame "Sample Start" {
                  n172 = local read "Command Start Readout"() -> (w113:u8[])
                  n173 = local read "Data Sample Start"() -> (w105:u8[])
                  n174 = Array Size(array=w105) -> (size(s)=w104:i32)
                  n175 = Index Array(array=w105, index=w106) -> (element=w112:u8)
                  n176 = Index Array(array=w113, index=w111) -> (element=w114:u8)
                  n177 = Replace Array Subset(array=w109, new element=w112, index=w106) -> (w107:u8[])
                  n178 = Replace Array Subset(array=w110, new element=w114, index=w111) -> (w108:u8[])
                }
                frame "Sample End" {
                  n179 = local read "Command End Readout"() -> (w124:u8[])
                  n180 = local read "Data Sample End"() -> (w116:u8[])
                  n181 = Array Size(array=w116) -> (size(s)=w115:i32)
                  n182 = Index Array(array=w116, index=w117) -> (element=w123:u8)
                  n183 = Index Array(array=w124, index=w122) -> (element=w125:u8)
                  n184 = Replace Array Subset(array=w120, new element=w123, index=w117) -> (w118:u8[])
                  n185 = Replace Array Subset(array=w121, new element=w125, index=w122) -> (w119:u8[])
                }
              }
              n186 = local write "Command"(w56) -> ()
              n187 = local write "Data"(w55) -> ()
              n188 = To Unsigned Byte Integer(number=w51) -> (unsigned 8bit integer=w52:u8)
              n189 = Less?(x=w51, y=w54) -> (x < y?=w53:bool)
              n190 = local write "ArraySize"(w52) -> ()
            }
            n191 = node-c288(w49) -> ()
            n192 = Not(x=w47) -> (.not. x?=w48:bool)
            n193 = local write "SetReg"(w48) -> ()
          }
        }
        "SetRegIsDone" <- w37
        n194 = local read "Stop_FPGA"() -> (w42:bool)
      }
      n195 = node-c288() -> (w13:T3)  [unwired: 1 in]
      n196 = while {
        shift-right: ["Конфигурация"] -> _
        shift-left: FALSE ("Конфигурация") -> [w133]
        stop <- w130 stop-if-true
        n197 = Greater?(x="Конфигурация", y=w133) -> (0:w132:bool)
        n198 = case shown="True" w132 {
          frame False {
            n199 = call "Wait2"("Count(Ticks)"=u8 2) -> ()  [unwired: 1 out]
          }
          frame True {
            n200 = call "ADC_spb.vi"(1:"18_1"=i8 18 ("18_1"), 2:"18_1"=i8 18 ("18_1"), "8"=i8 8, "7"=i8 7, "Write Data"="Write Data", "Enum"="Enum", "Read(T)/Write(F)"="Read(T)/Write(F)", "Command array"="Command array") -> ("READ"=→"READ":bool[])
          }
        }
        n201 = local read "Stop_FPGA"() -> (w130:bool)
      }
      n202 = timed-loop {
        timing: w13 -> [_]
        timing-out: [_] -> w12
        stop <- w27 stop-if-true
        # "IN1\tIN2\t\n\t0\t0\tOutTop_n\n\t0\t1\tOutTop_p\n\t1\t0\tOutBot_p\n\t1\t1\tOutBot_n"
        # "RS"
        # "CSBot"
        # "CSTop"
        # "IN1"
        # "IN2"
        n203 = xnode "FPGA I/O Node"("IO Module\\DDCA_DIO13_Write"="IN1") -> ()  [unwired: 1 in, 1 out]
        n204 = xnode "FPGA I/O Node"("IO Module\\DDCA_DIO14_Write"="IN2") -> ()  [unwired: 1 in, 1 out]
        n205 = xnode "FPGA I/O Node"("IO Module\\DDCA_DIO16_Write"="CSTop") -> ()  [unwired: 1 in, 1 out]
        n206 = xnode "FPGA I/O Node"("IO Module\\DDCA_DIO20_Write"="CSBot") -> ()  [unwired: 1 in, 1 out]
        n207 = xnode "FPGA I/O Node"("IO Module\\DDCA_DIO23_Write"="RS") -> ()  [unwired: 1 in, 1 out]
        n208 = local read "Stop_FPGA"() -> (w27:bool)
      }
      n209 = node-c288(w12) -> ()
      n210 = node-c288(w25) -> ()
    }
  }
